vi "create swept sine wavepackets (SubVI).vi"(6 "Cluster":T1, 7 "center freq [MHz]":dbl, 8 "calib(F)/monitor(T)":bool, 9 "sampling period [us] in":dbl, 10 "delay [us]":dbl, 11 "voltage range [470-1450mV]":dbl) -> (2 "Array":dbl[](array[numeric]), 3 "Numeric":u32)   [LabVIEW 2024]
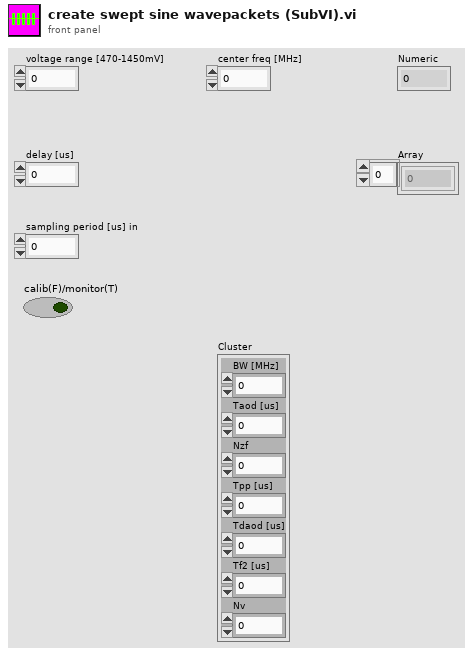
[diagram p1: front panel]
types:
  T1 = cluster{"BW [MHz]":dbl, "Taod [us]":dbl, "Nzf":i32, "Tpp [us]":dbl, "Tdaod [us]":dbl, "Tf2 [us]":dbl, "Nv":dbl}
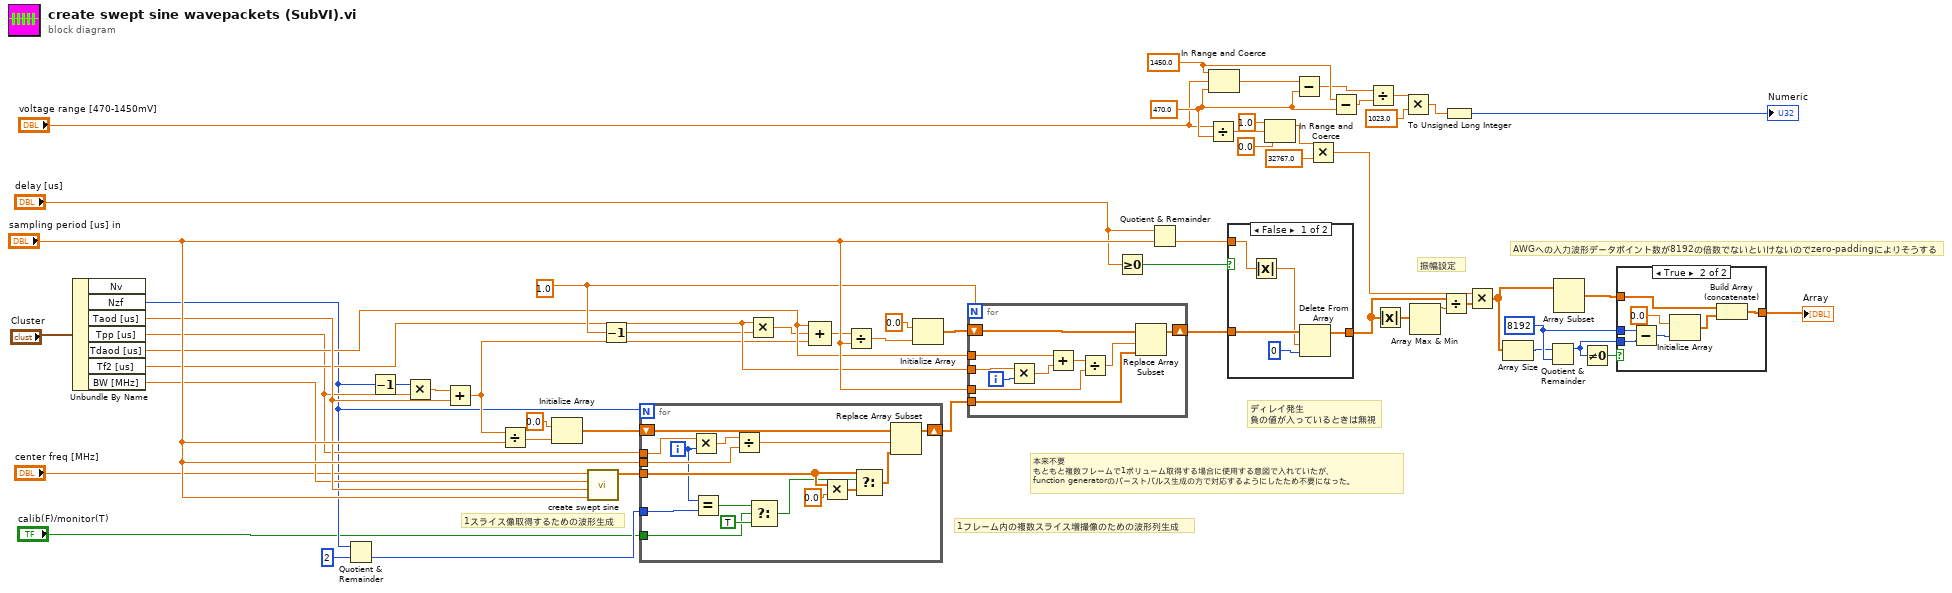
[diagram p0: block diagram]
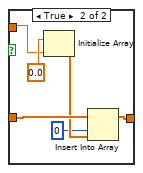
[diagram p2: hidden frame]
diagram:
  w55 = 1.0
  w18 = 1450.0 ("x")
  w20 = 470.0 ("y")
  w9 = 8192 ("y")
  # "AWGへの入力波形データポイント数が8192の倍数でないといけないのでzero-paddingによりそうする"
  # "振幅設定"
  # "ディレイ発生\n負の値が入っているときは無視"
  # "1スライス像取得するための波形生成"
  # "1フレーム内の複数スライス増撮像のための波形列生成"
  # "本来不要\nもともと複数フレームで1ボリューム取得する場合に使用する意図で入れていたが、\nfunction generatorのバーストパルス生成の方で対応するようにしたため不要になった。"
  n1 = Unbundle By Name("Cluster") -> ("Nzf"=w4:i32, "Taod [us]"=w53:dbl, "Tpp [us]"=w44:dbl, "Tdaod [us]"=w45:dbl, "Tf2 [us]"=w46:dbl, "BW [MHz]"=w43:dbl)  [unwired: 1 out]
  n2 = Quotient & Remainder(x=w4, y=2) -> (floor(x/y)=w2:i32)  [unwired: 1 out]
  n3 = Decrement(x=w4) -> (x-1=w33:i32)
  n4 = Multiply(x=w33, y=w44) -> (x*y=w34:dbl)
  n5 = Add(x=w34, y=w53) -> (x+y=w38:dbl)
  n6 = Divide(x=w38, y="sampling period [us] in") -> (x/y=w36:dbl)
  n7 = Initialize Array(0.0 ("element"), w36) -> (w37:dbl[])
  n8 = call "create swept sine.vi"("sampling period [us] in"="sampling period [us] in", "duration [us]"=w53, "bandwidth [MHz]"=w43, "center freq [MHz]"="center freq [MHz]") -> ("waveform"=w27:dbl[])  [unwired: 6 in, 1 out]
  n9 = Decrement(x=w55) -> (x-1=w28:dbl)
  n10 = for {
    N: w4 -> [_]
    tunnel: w27 -> [w66]
    shift-right: [w72] -> w54
    shift-left: w37 -> [w73]
    tunnel: w44 -> [w74]
    tunnel: "sampling period [us] in" -> [w70]
    tunnel: w2 -> [w63]
    tunnel: "calib(F)/monitor(T)" -> [w59]
    i -> [w64]
    n11 = Multiply(x=w74, y=w64) -> (x*y=w71:dbl)
    n12 = Equal?(x=w64, y=w63) -> (x = y?=w62:bool)
    n13 = Divide(x=w71, y=w70) -> (x/y=w69:dbl)
    n14 = Select(t=w62, s=w59, f=TRUE) -> (s? t:f=w61:bool)
    n15 = Multiply(x=w66, y=0.0) -> (x*y=w67:dbl[])
    n16 = Select(t=w66, s=w61, f=w67) -> (s? t:f=w65:dbl[])
    n17 = Replace Array Subset(array=w73, new element=w65, index=w69) -> (w72:dbl[])
  }
  n18 = Multiply(x=w46, y=w28) -> (x*y=w29:dbl)
  n19 = Compound Arithmetic op=ADD(w45, w29, w38) -> (w30:dbl)
  n20 = Divide(x=w30, y="sampling period [us] in") -> (x/y=w31:dbl)
  n21 = Initialize Array(0.0 ("element"), w31) -> (w39:dbl[])
  n22 = for {
    N: w55 -> [_]
    shift-right: [w76] -> w48
    shift-left: w39 -> [w77]
    tunnel: w46 -> [w84]
    tunnel: w45 -> [w81]
    tunnel: "sampling period [us] in" -> [w79]
    tunnel: w54 -> [w78]
    i -> [w83]
    n23 = Multiply(x=w84, y=w83) -> (x*y=w82:dbl)
    n24 = Add(x=w81, y=w82) -> (x+y=w80:dbl)
    n25 = Divide(x=w80, y=w79) -> (x/y=w75:dbl)
    n26 = Replace Array Subset(array=w77, new element=w78, index=w75) -> (w76:dbl[])
  }
  n27 = Greater Or Equal To 0?(x="delay [us]") -> (x >= 0?=w52:bool)
  n28 = Quotient & Remainder(x="delay [us]", y="sampling period [us] in") -> (floor(x/y)=w51:dbl)  [unwired: 1 out]
  n29 = Divide(x="voltage range [470-1450mV]", y=w20) -> (x/y=w22:dbl)
  n30 = In Range and Coerce(upper limit=w18, x="voltage range [470-1450mV]", lower limit=w20) -> (coerced(x)=w17:dbl)  [unwired: 1 out]
  n31 = case shown="False" w52 {
    tunnel: w48 -> [w88 w95]
    tunnel: [w85 w91] -> w49
    tunnel: w51 -> [w87 w93]
    frame False {
      n32 = Absolute Value(x=w87) -> (abs(x)=w86:dbl)
      n33 = Delete From Array(array=w88, length=w86, index=0) -> (array with subset deleted=w85:dbl[])  [unwired: 1 out]
    }
    frame True {
      n34 = Initialize Array(0.0 ("element"), w93) -> (w92:dbl[])
      n35 = Insert Into Array(array=w95, index=0, new element=w92) -> (w91:dbl[])
    }
  }
  n36 = In Range and Coerce(upper limit=1.0, x=w22, lower limit=0.0) -> (coerced(x)=w25:dbl)  [unwired: 1 out]
  n37 = Subtract(x=w17, y=w20) -> (x-y=w12:dbl)
  n38 = Multiply(x=w25, y=32767.0) -> (x*y=w26:dbl)
  n39 = Subtract(x=w18, y=w20) -> (x-y=w13:dbl)
  n40 = Divide(x=w12, y=w13) -> (x/y=w14:dbl)
  n41 = Absolute Value(x=w49) -> (abs(x)=w40:dbl[])
  n42 = Multiply(x=w14, y=1023.0) -> (x*y=w16:dbl)
  n43 = Array Max & Min(array=w40) -> (max value=w10:dbl)  [unwired: 3 out]
  n44 = Divide(x=w49, y=w10) -> (x/y=w11:dbl[])
  n45 = To Unsigned Long Integer(number=w16) -> (unsigned 32bit integer=→"Numeric":u32)
  n46 = Multiply(x=w26, y=w11) -> (x*y=w41:dbl[])
  n47 = Array Size(array=w41) -> (size(s)=w5:i32)
  n48 = Quotient & Remainder(x=w5, y=w9) -> (x-y*floor(x/y)=w7:i32)  [unwired: 1 out]
  n49 = Array Subset(array=w41) -> (w8:dbl[])  [unwired: 2 in]
  n50 = Not Equal To 0?(x=w7) -> (x != 0?=w6:bool)
  n51 = case shown="True" w6 {
    tunnel: w8 -> [w96 w97]
    tunnel: [w96 w101] -> w57
    tunnel: w7 -> [_ w99]
    tunnel: w9 -> [_ w100]
    frame False {
    }
    frame True {
      n52 = Subtract(x=w100, y=w99) -> (x-y=w98:i32)
      n53 = Initialize Array(0.0 ("element"), w98) -> (w102:dbl[])
      n54 = Build Array (concatenate)(w97, w102) -> (w101:dbl[])
    }
  }
  "Array" <- w57
